vi "SegmentsFinalize_171213.vi"(6 "BorderColor":u32[](array[numeric]), 9 "MidfieldColor":u32[](array[numeric]), 10 "CenterColor":u32[](array[numeric]), 11 "InputBackground":picture) -> (1 "TotalNumberOfSegments":i32, 2 "RegionNameList":string[](array[string]), 3 "Outputbackground":picture, 4 "OutputPixmapforEvents":u32[][](array[numeric]), 5 "ColorArrayforEvents":u32[](array[numeric]))   [LabVIEW 2016]
uses:
  Globaltracker.vi
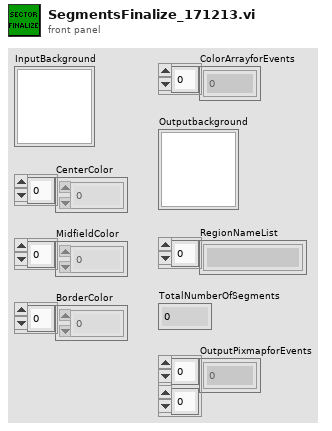
[diagram p1: front panel]
types:
  T1 = typedef "imagedata.ctl" = cluster{"image type":i32, "image depth":i32, "image":u8[], "mask":u8[], "colors":u32[], "Rectangle":cluster{"left":i16, "top":i16, "right":i16, "bottom":i16}}
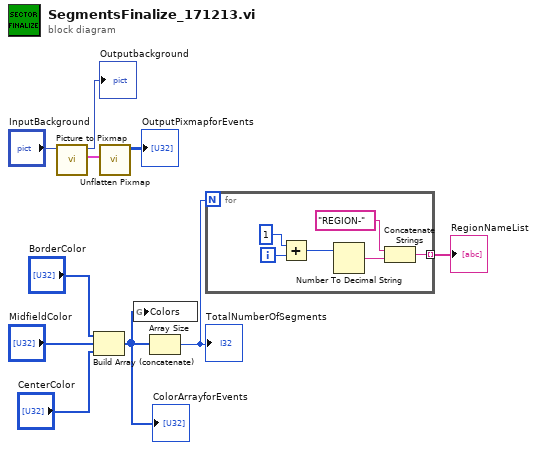
[diagram p0: block diagram]
diagram:
  n1 = call <vilib>:"Picture to Pixmap.vi"("picture"="InputBackground") -> ("image data"=w1:T1, "new picture"=→"Outputbackground":picture)  [unwired: 9 in]
  n2 = Build Array (concatenate)("BorderColor", "MidfieldColor", "CenterColor") -> (w8:u32[])
  "ColorArrayforEvents" <- w8
  n3 = call <vilib>:"Unflatten Pixmap.vi"("image data"=w1) -> ("24-bit pixmap"=→"OutputPixmapforEvents":u32[][])  [unwired: 4 in, 6 out]
  n4 = global write "Globaltracker.vi" "Colors"(w8) -> ()
  n5 = Array Size(array=w8) -> (size(s)=w7:i32)
  "TotalNumberOfSegments" <- w7
  n6 = for {
    N: w7 -> [_]
    tunnel: [w11] -> w6 mode=indexing
    i -> [w15]
    n7 = Add(x=1, y=w15) -> (x+y=w13:i32)
    n8 = Number To Decimal String(number=w13) -> (decimal integer string=w12:string)  [unwired: 1 in]
    n9 = Concatenate Strings("REGION-", w12) -> (w11:string)
  }
  "RegionNameList" <- w6
